vi "Do Request.vi"(7 "Inputs":T2, 8 "error in (no error)":errorcluster, 11 "Test Sessions Controller in":refnum<class "Test Sessions Controller.lvclass">) -> (0 "error out":errorcluster, 5 "Outputs":T1)   [LabVIEW 2020, in "Test Sessions Controller.lvclass"]
uses:
  Test Sessions Controller.lvclass
  HTTP Server/Controller Inputs.ctl
  HTTP Server/Values/Values.lvclass
  <vilib>/IlluminatedG/IG HTTP Utils/HTTP Utils/Request/Request.lvclass
  HTTP Server/Session/Session.lvclass
  HTTP Server/Controller Outputs.ctl
  <vilib>/IlluminatedG/IG HTTP Utils/HTTP Utils/Response/Response.lvclass
  <vilib>/IlluminatedG/lv-stream/URI/URI.lvclass
  HTTP Server/HTTP Server.lvlib
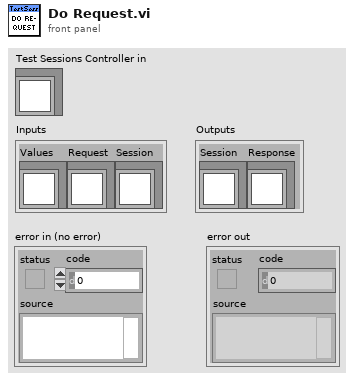
[diagram p1: front panel]
types:
  T1 = typedef "HTTP Server.lvlib/Controller Outputs.ctl" = cluster{"Session":refnum<class "Session.lvclass">, "Response":refnum<class "Response.lvclass">}
  T2 = typedef "HTTP Server.lvlib/Controller Inputs.ctl" = cluster{"Values":refnum<class "Values.lvclass">, "Request":refnum<class "Request.lvclass">, "Session":refnum<class "Session.lvclass">}
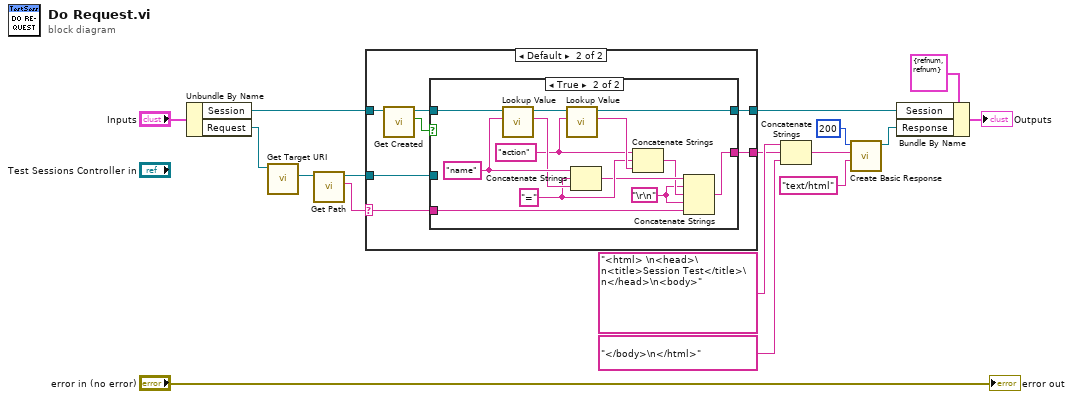
[diagram p0: block diagram]
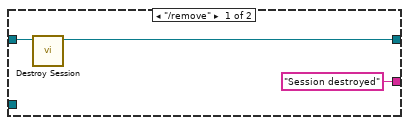
[diagram p2: hidden frame]
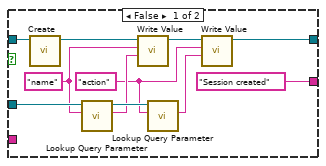
[diagram p3: hidden frame]
diagram:
  n1 = Unbundle By Name("Inputs") -> ("Session"=w15:refnum<class "Session.lvclass">, "Request"=w14:refnum<class "Request.lvclass">)
  n2 = call <vilib>:"Get Target URI.vi"("Request in"=w14) -> ("Target URI"=w13:refnum<class "URI.lvclass">)  [unwired: 8 in, 2 out]
  n3 = call <vilib>:"Get Path.vi"("URI in"=w13) -> ("Path"=w11:string, "URI out"=w12:refnum<class "URI.lvclass">)  [unwired: 8 in, 1 out]
  n4 = case shown="Default" w11 {
    selector: w11 -> [_ w21]
    tunnel: w15 -> [w19 w27]
    tunnel: w12 -> [_ w24]
    tunnel: [w18 w23] -> w3
    tunnel: ["Session destroyed" ("Name") w22] -> w5
    frame "/remove" {
      n5 = call "Destroy Session.vi"("Session in"=w19) -> ("Session out"=w18:refnum<class "Session.lvclass">)  [unwired: 9 in, 1 out]
    }
    frame Default {
      n6 = call "Get Created.vi"("Session in"=w27) -> ("Created"=w26:bool, "Session out"=w25:refnum<class "Session.lvclass">)  [unwired: 8 in, 1 out]
      n7 = case shown="True" w26 {
        tunnel: w25 -> [w36 w51]
        tunnel: w24 -> [w38 _]
        tunnel: [w29 w49] -> w23
        tunnel: ["Session created" ("Name") w41] -> w22
        tunnel: w21 -> [_ w39]
        frame False {
          w30 = "action" ("Name")
          w34 = "name" ("Name")
          n8 = call "Create.vi"("Session in"=w36) -> ("Session out"=w35:refnum<class "Session.lvclass">)  [unwired: 9 in, 1 out]
          n9 = call <vilib>:"Lookup Query Parameter.vi"("Name"=w34, "URI in"=w38) -> ("Value"=w33:string, "URI out"=w37:refnum<class "URI.lvclass">)  [unwired: 6 in, 2 out]
          n10 = call "Write Value.vi"("Value"=w33, "Name"=w34, "Session in"=w35) -> ("Session out"=w32:refnum<class "Session.lvclass">)  [unwired: 6 in, 2 out]
          n11 = call <vilib>:"Lookup Query Parameter.vi"("Name"=w30, "URI in"=w37) -> ("Value"=w31:string)  [unwired: 6 in, 3 out]
          n12 = call "Write Value.vi"("Value"=w31, "Name"=w30, "Session in"=w32) -> ("Session out"=w29:refnum<class "Session.lvclass">)  [unwired: 6 in, 2 out]
        }
        frame True {
          w40 = "\r\n"
          w44 = "=" ("string")
          w45 = "action" ("Name")
          w48 = "name" ("Name")
          n13 = call "Lookup Value.vi"("Name"=w48, "Session in"=w51) -> ("Value"=w47:string, "Session out"=w50:refnum<class "Session.lvclass">)  [unwired: 6 in, 2 out]
          n14 = call "Lookup Value.vi"("Name"=w45, "Session in"=w50) -> ("Value"=w46:string, "Session out"=w49:refnum<class "Session.lvclass">)  [unwired: 6 in, 2 out]
          n15 = Concatenate Strings(w48, w44, w47) -> (w43:string)
          n16 = Concatenate Strings(w45, w44, w46) -> (w42:string)
          n17 = Concatenate Strings(w43, w40, w42, w40, w39) -> (w41:string)
        }
      }
    }
  }
  n18 = Concatenate Strings("<html> \n<head>\n<title>Session Test</title>\n</head>\n<body>", w5, "</body>\n</html>") -> (w6:string)
  n19 = call <vilib>:"Create Basic Response.vi"("Content-Type (text/plain)"="text/html", "Payload"=w6, "Status Code"=u16 200) -> ("Response out"=w2:refnum<class "Response.lvclass">)  [unwired: 7 in, 1 out]
  n20 = Bundle By Name(cluster=T1 {"Session"=refnum, "Response"=refnum} ("Outputs"), "Session"=w3, "Response"=w2) -> (→"Outputs":T1)
  "error out" <- "error in (no error)"
